vi "util_InitializeTable.vi"(6 "error in":errorcluster, 7 "Reset Filter Wheels":bool=TRUE) -> (0 "Status Cluster":T1, 1 "Success":bool, 2 "error out":errorcluster, 3 "FPGA VI Reference Out":refnum<k20>)   [LabVIEW 2012]
uses:
  <vilib>/Utility/error.llb/DialogType.ctl
  <vilib>/FPGAPlugInAG/PCIe-7841R/niLvFpga_Open_PCIe-7841R.vi
  <vilib>/rvi/interface/common/dynamic/niFpgaDynamicAddResources.vi
  <vilib>/Utility/error.llb/Error Cluster From Error Code.vi
  <vilib>/rvi/errors/niLvFpgaAdjustHostInterfaceError.vi
  <vilib>/rvi/interface/nirviOpenFPGA/nirviOpenFPGA.xnode
  FPGA Bitfiles/OptogeneticsTabl_FPGATarget_OpticsIO(FPGA)_9A6V+shJCSE.lvbitx
  OpticsIO (FPGA).vi
  <vilib>/rvi/interface/nirviReadWriteControl/nirviReadWriteControl.xnode
  NiFpgaLv.dll
  <vilib>/rvi/interface/Simulation/niFpgaSimulationCallBeginRW.vi
panel:
  in  "Scaffold":T1
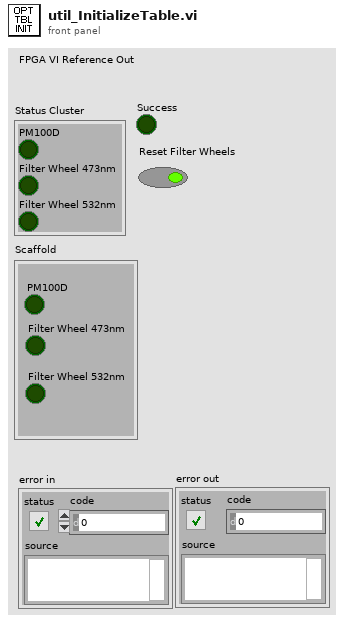
[diagram p1: front panel]
types:
  T1 = cluster{"PM100D":bool, "Filter Wheel 473nm":bool, "Filter Wheel 532nm":bool}
  T2 = cluster{"Pulse Length (Ticks)":u32, "Pulse Period (Ticks)":u32, "Ao (Int)":i32, "Seq 1 (High)":bool, "Seq 2 (Low)":bool}
  T3 = typedef "DialogType.ctl" = u16
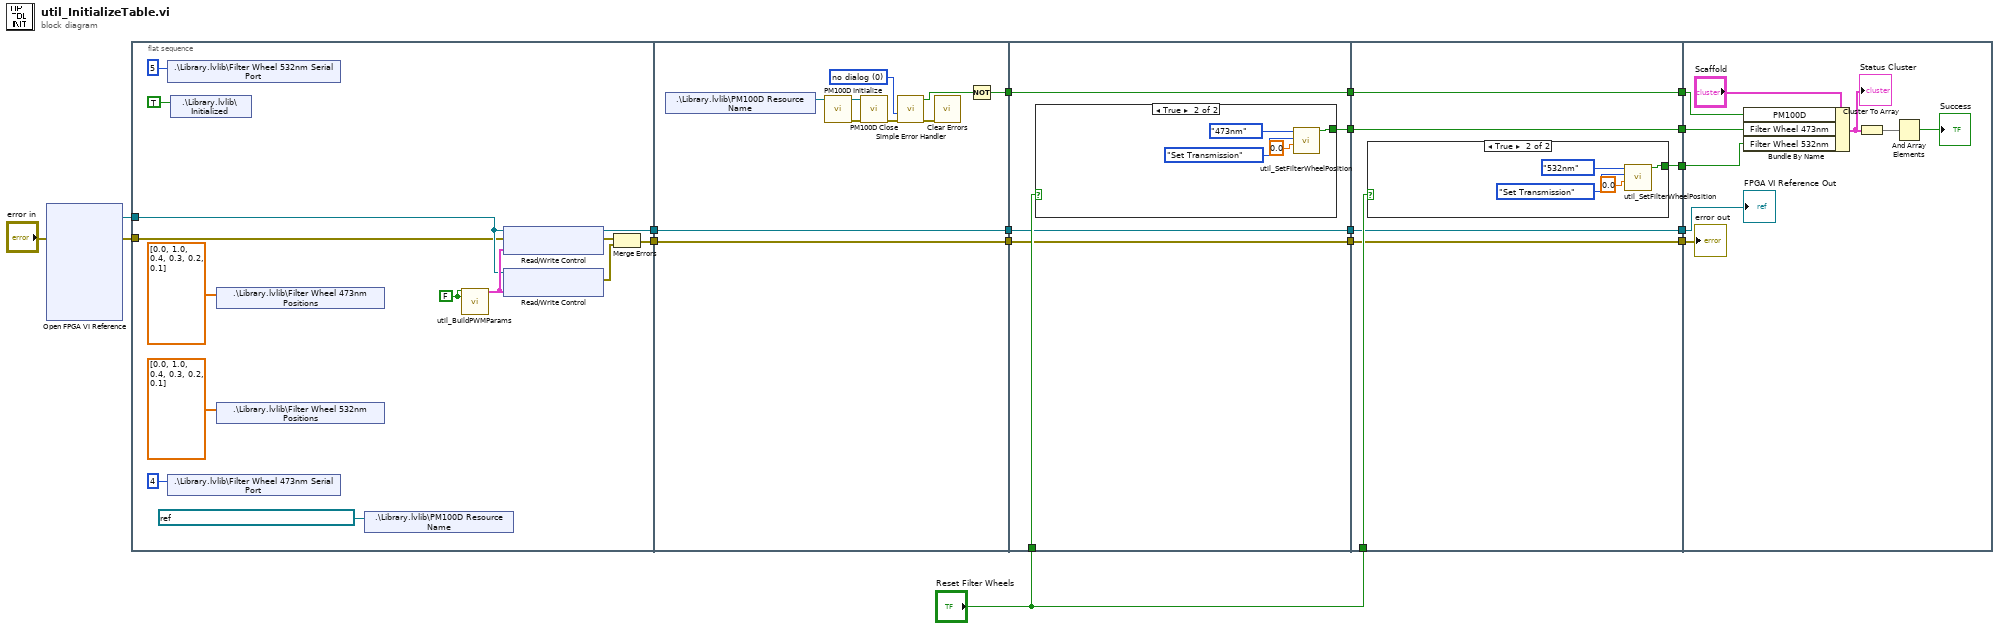
[diagram p0: block diagram]
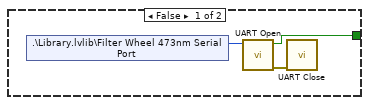
[diagram p2: hidden frame]
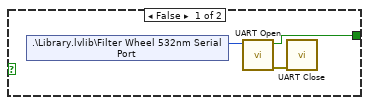
[diagram p3: hidden frame]
diagram:
  n1 = xnode "Open FPGA VI Reference"("error in"="error in") -> ("FPGA VI Reference Out"=w11:refnum<k20>, "error out"=w6:errorcluster)  [unwired: 1 in]
  n2 = flat-sequence {
    tunnel: w11 -> [w24]
    tunnel: [w23] -> w7
    tunnel: w6 -> [w22]
    tunnel: [w19] -> w4
    tunnel: [w39] -> w15
    tunnel: [w34] -> w10
    tunnel: w7 -> [w34]
    tunnel: [w33] -> w5
    tunnel: w4 -> [w33]
    tunnel: [w47] -> w16
    tunnel: w15 -> [w47]
    tunnel: "Reset Filter Wheels" -> [w46]
    tunnel: [w45] -> w12
    tunnel: w10 -> [w44]
    tunnel: [w44] -> w9
    tunnel: w5 -> [w43]
    tunnel: [w43] -> w2
    tunnel: [w57] -> w18
    tunnel: [w60] -> w17
    tunnel: w16 -> [w60]
    tunnel: "Reset Filter Wheels" -> [w58]
    tunnel: [w59] -> w13
    tunnel: w12 -> [w59]
    tunnel: w9 -> [w56]
    tunnel: [w56] -> w8
    tunnel: [w55] -> w3
    tunnel: w2 -> [w55]
    tunnel: w18 -> [w74]
    tunnel: w17 -> [w75]
    tunnel: w13 -> [w70]
    tunnel: w8 -> [w69]
    tunnel: w3 -> [w68]
    frame #0 {
      w26 = FALSE ("Burst")
      n3 = shared-variable ".\\Library.lvlib\\Filter Wheel 532nm Serial Port"(i8 5 ("Filter Wheel 532nm Serial Port")) -> ()  [unwired: 1 in, 1 out]
      n4 = shared-variable ".\\Library.lvlib\\Filter Wheel 473nm Serial Port"(i8 4 ("Filter Wheel 532nm Serial Port")) -> ()  [unwired: 1 in, 1 out]
      n5 = shared-variable ".\\Library.lvlib\\Initialized"(TRUE ("Initialized")) -> ()  [unwired: 1 in, 1 out]
      n6 = shared-variable ".\\Library.lvlib\\Filter Wheel 473nm Positions"(dbl[] [0.0, 1.0, 0.4, 0.3, 0.2, 0.1]) -> ()  [unwired: 1 in, 1 out]
      n7 = shared-variable ".\\Library.lvlib\\Filter Wheel 532nm Positions"(dbl[] [0.0, 1.0, 0.4, 0.3, 0.2, 0.1]) -> ()  [unwired: 1 in, 1 out]
      n8 = shared-variable ".\\Library.lvlib\\PM100D Resource Name"(refnum<visa-resource-name> "USB0::0x1313::0x8078::P0006758::INSTR" ("PM100D Resource Name")) -> ()  [unwired: 1 in, 1 out]
      n9 = call "util_BuildPWMParams.vi"("Burst"=w26, "Continous"=w26) -> ("PWM Params"=w25:T2)  [unwired: 13 in]
      n10 = xnode "Read/Write Control"("FPGA VI Reference In"=w24, "error in"=w22, "PWM 532nm Laser"=w25) -> ("FPGA VI Reference Out"=w23:refnum<k20>, "error out"=w21:errorcluster)
      n11 = xnode "Read/Write Control"("FPGA VI Reference In"=w24, "PWM 473nm Laser"=w25) -> ("error out"=w20:errorcluster)  [unwired: 1 in, 1 out]
      n12 = Merge Errors(w21, w20) -> (w19:errorcluster)
    }
    frame #1 {
      w42 = T3 0 items=["no dialog", "OK message", "continue or stop message", "OK message + warnings", "continue/stop + warnings"] ("type of dialog (OK msg:1)")
      n13 = shared-variable ".\\Library.lvlib\\PM100D Resource Name"() -> (w38:refnum<visa-resource-name>)  [unwired: 1 in, 1 out]
      n14 = call <instrlib>:"PM100D Initialize.vi"("resource name"=w38) -> ("error out"=w36:errorcluster, "instrument handle out"=w37:refnum<visa-resource-name>)  [unwired: 9 in]
      n15 = call <instrlib>:"PM100D Close.vi"("error in (no error)"=w36, "instrument handle"=w37) -> ("error out"=w35:errorcluster)  [unwired: 9 in]
      n16 = call <vilib>:"Simple Error Handler.vi"("type of dialog (OK msg:1)"=w42, "error in (no error)"=w35) -> ("error?"=w40:bool, "error out"=w41:errorcluster)  [unwired: 3 in, 3 out]
      n17 = call <vilib>:"Clear Errors.vi"("error in (no error)"=w41) -> ()  [unwired: 6 in, 1 out]
      n18 = Not(x=w40) -> (.not. x?=w39:bool)
    }
    frame #2 {
      n19 = case shown="True" w46 {
        tunnel: [w48 w51] -> w45
        frame False {
          n20 = shared-variable ".\\Library.lvlib\\Filter Wheel 473nm Serial Port"() -> (w50:i8)  [unwired: 1 in, 1 out]
          n21 = call "UART Open.vi"("Serial Port"=w50) -> ("error out"=w49:errorcluster, "Success?"=w48:bool)  [unwired: 9 in]
          n22 = call "UART Close.vi"("error in (no error)"=w49) -> ()  [unwired: 10 in, 1 out]
        }
        frame True {
          n23 = call "util_SetFilterWheelPosition.vi"("Filter Transmission"=0.0, "Mode"=enum16{"Set Position", "Set Transmission"}."Set Transmission", "Filter Wheel"=enum16{"473nm", "532nm"}."473nm") -> ("Success"=w51:bool)  [unwired: 8 in]
        }
      }
    }
    frame #3 {
      n24 = case shown="True" w58 {
        tunnel: [w62 w64] -> w57
        frame False {
          n25 = shared-variable ".\\Library.lvlib\\Filter Wheel 532nm Serial Port"() -> (w63:i8)  [unwired: 1 in, 1 out]
          n26 = call "UART Open.vi"("Serial Port"=w63) -> ("error out"=w61:errorcluster, "Success?"=w62:bool)  [unwired: 9 in]
          n27 = call "UART Close.vi"("error in (no error)"=w61) -> ()  [unwired: 10 in, 1 out]
        }
        frame True {
          n28 = call "util_SetFilterWheelPosition.vi"("Filter Transmission"=0.0, "Mode"=enum16{"Set Position", "Set Transmission"}."Set Transmission", "Filter Wheel"=enum16{"473nm", "532nm"}."532nm") -> ("Success"=w64:bool)  [unwired: 8 in]
        }
      }
    }
    frame #4 {
      n29 = Bundle By Name(cluster="Scaffold", "PM100D"=w75, "Filter Wheel 473nm"=w70, "Filter Wheel 532nm"=w74) -> (w71:T1)
      "Status Cluster" <- w71
      n30 = Cluster To Array(cluster=w71) -> (array=w73:bool[])
      n31 = And Array Elements(Boolean array=w73) -> (logical AND=→"Success":bool)
      "FPGA VI Reference Out" <- w69
      "error out" <- w68
    }
  }
